vi "Get Network Endpoint Enqueuer.vi"(8 "error in":errorcluster, 11 "MSS Target Actor in":refnum<class "MSS Target Actor.lvclass">) -> (0 "error out":errorcluster, 2 "Enqueuer":refnum<class "Message Enqueuer.lvclass">, 3 "MSS Target Actor out":refnum<class "MSS Target Actor.lvclass">)   [LabVIEW 2023, in "MSS Target Actor.lvlib" / "MSS Target Actor.lvclass"]
uses:
  MSS Target Actor.lvclass
  MSS Target Actor.lvclass/MSS Target Actor.ctl
  <vilib>/ErrorRing/Error Ring.xnode
  <vilib>/Utility/error.llb/Error Cluster From Error Code.vi
  <vilib>/ActorFramework/Message Enqueuer/Message Enqueuer.lvclass
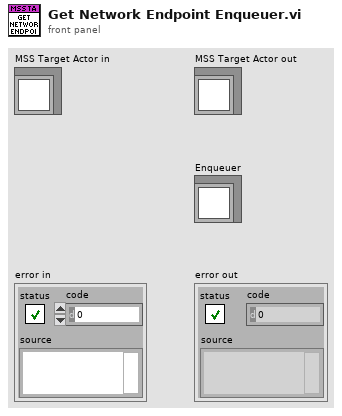
[diagram p1: front panel]
types:
  T1 = map{string, refnum<class "Message Enqueuer.lvclass">}
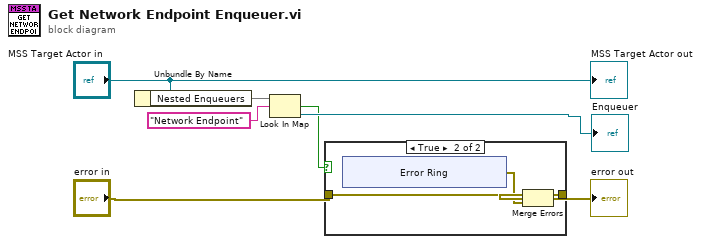
[diagram p0: block diagram]
diagram:
  n1 = Unbundle By Name("MSS Target Actor in") -> ("Nested Enqueuers"=w3:T1)
  n2 = Look In Map(map=w3, key="Network Endpoint") -> (key not found?=w1:bool, value=→"Enqueuer":refnum<class "Message Enqueuer.lvclass">)  [unwired: 1 in]
  n3 = case shown="True" w1 {
    tunnel: "error in" -> [w8 w11]
    tunnel: [w8 w10] -> w6
    frame False {
    }
    frame True {
      n4 = xnode "Error Ring"() -> ("error out"=w9:errorcluster)
      n5 = Merge Errors(w11, w9) -> (w10:errorcluster)
    }
  }
  "error out" <- w6
  "MSS Target Actor out" <- "MSS Target Actor in"
